vi "15.10.04 Interface+Data1.vi"() -> ()   [LabVIEW 2014]
panel:
  in  "NÚMERO DE CICLOS":dbl
  in  "Liga/Desliga":bool
  in  "Escolha: Porta Serial":refnum<visa-resource-name>="COM3"
  out "Dessorção":bool
  out "Adssorção":bool
  out "Single-Pass":bool
  out "Batch":bool
  in  "BATCH / SINGLE PASS":bool
  in  "Corrente":path
  in  "pH":path
  in  "Condutividade":path
  out "CORRENTE (A)":dbl(graph)
  out "pH":dbl(graph)
  out "CONDUTIVIDADE (us/cm)":dbl(graph)
  in  "?":enum32{"POTENCIOSTÁTICO", "GALVANOSTÁTICO"}(tab)
  in  "CONDUTIVIDADE \nMÁXIMA NA DESSORÇÃO P":dbl
  in  "TEMPO DE DESSOR敲O P":dbl
  in  "CONDUTIVIDADE \nMÍNIMA NA ADSORÇÃO P":dbl
  in  "TEMPO DE ADSOR敲O P":dbl
  in  "POTENCIAL DE CORTE\nNA DESSOR敲O (V) G":dbl
  in  "POTENCIAL DE CORTE\nNA ADSOR敲O (V) G":dbl
  in  "CONDUTIVIDADE \nMÍNIMA NA DESSORÇÃO G":dbl
  in  "TEMPO DE DESSOR敲O G":dbl
  in  "CONDUTIVIDADE \nMÍNIMA NA ADSORÇÃO G":dbl
  in  "TEMPO DE ADSOR敲O G":dbl
  # "s"
  # "us/cm"
  # "s"
  # "us/cm"
  # "s"
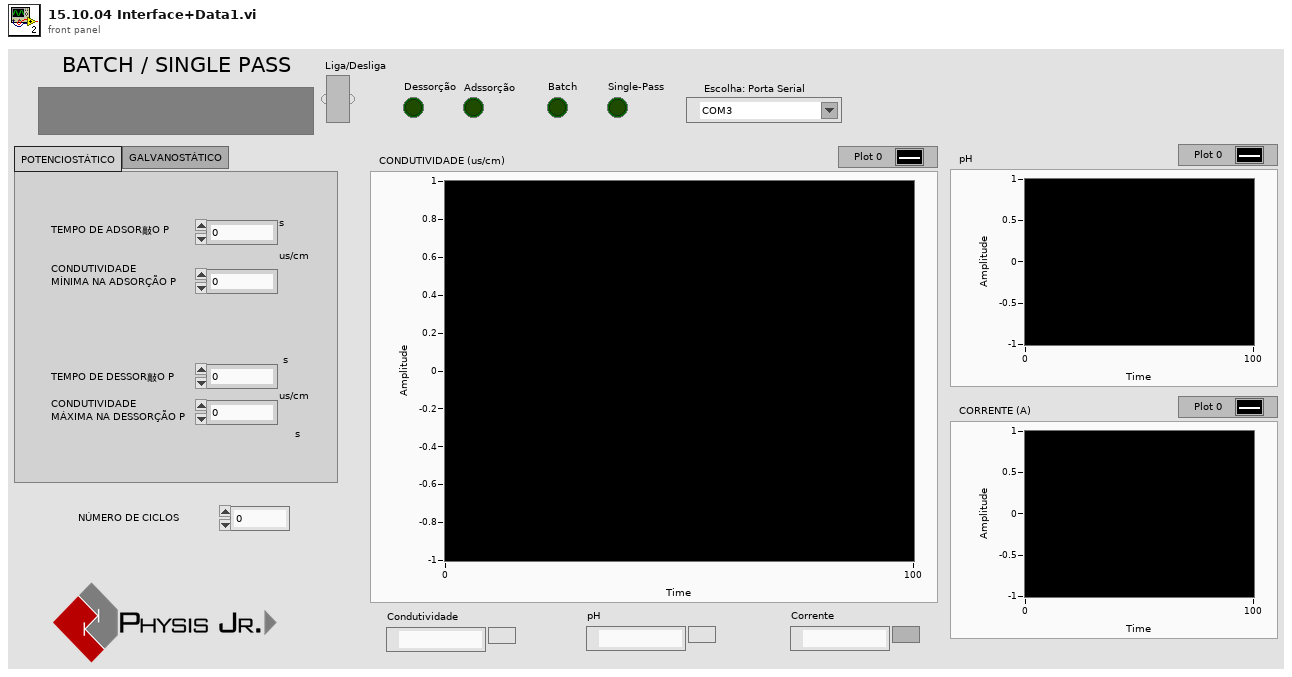
[diagram p1: front panel]
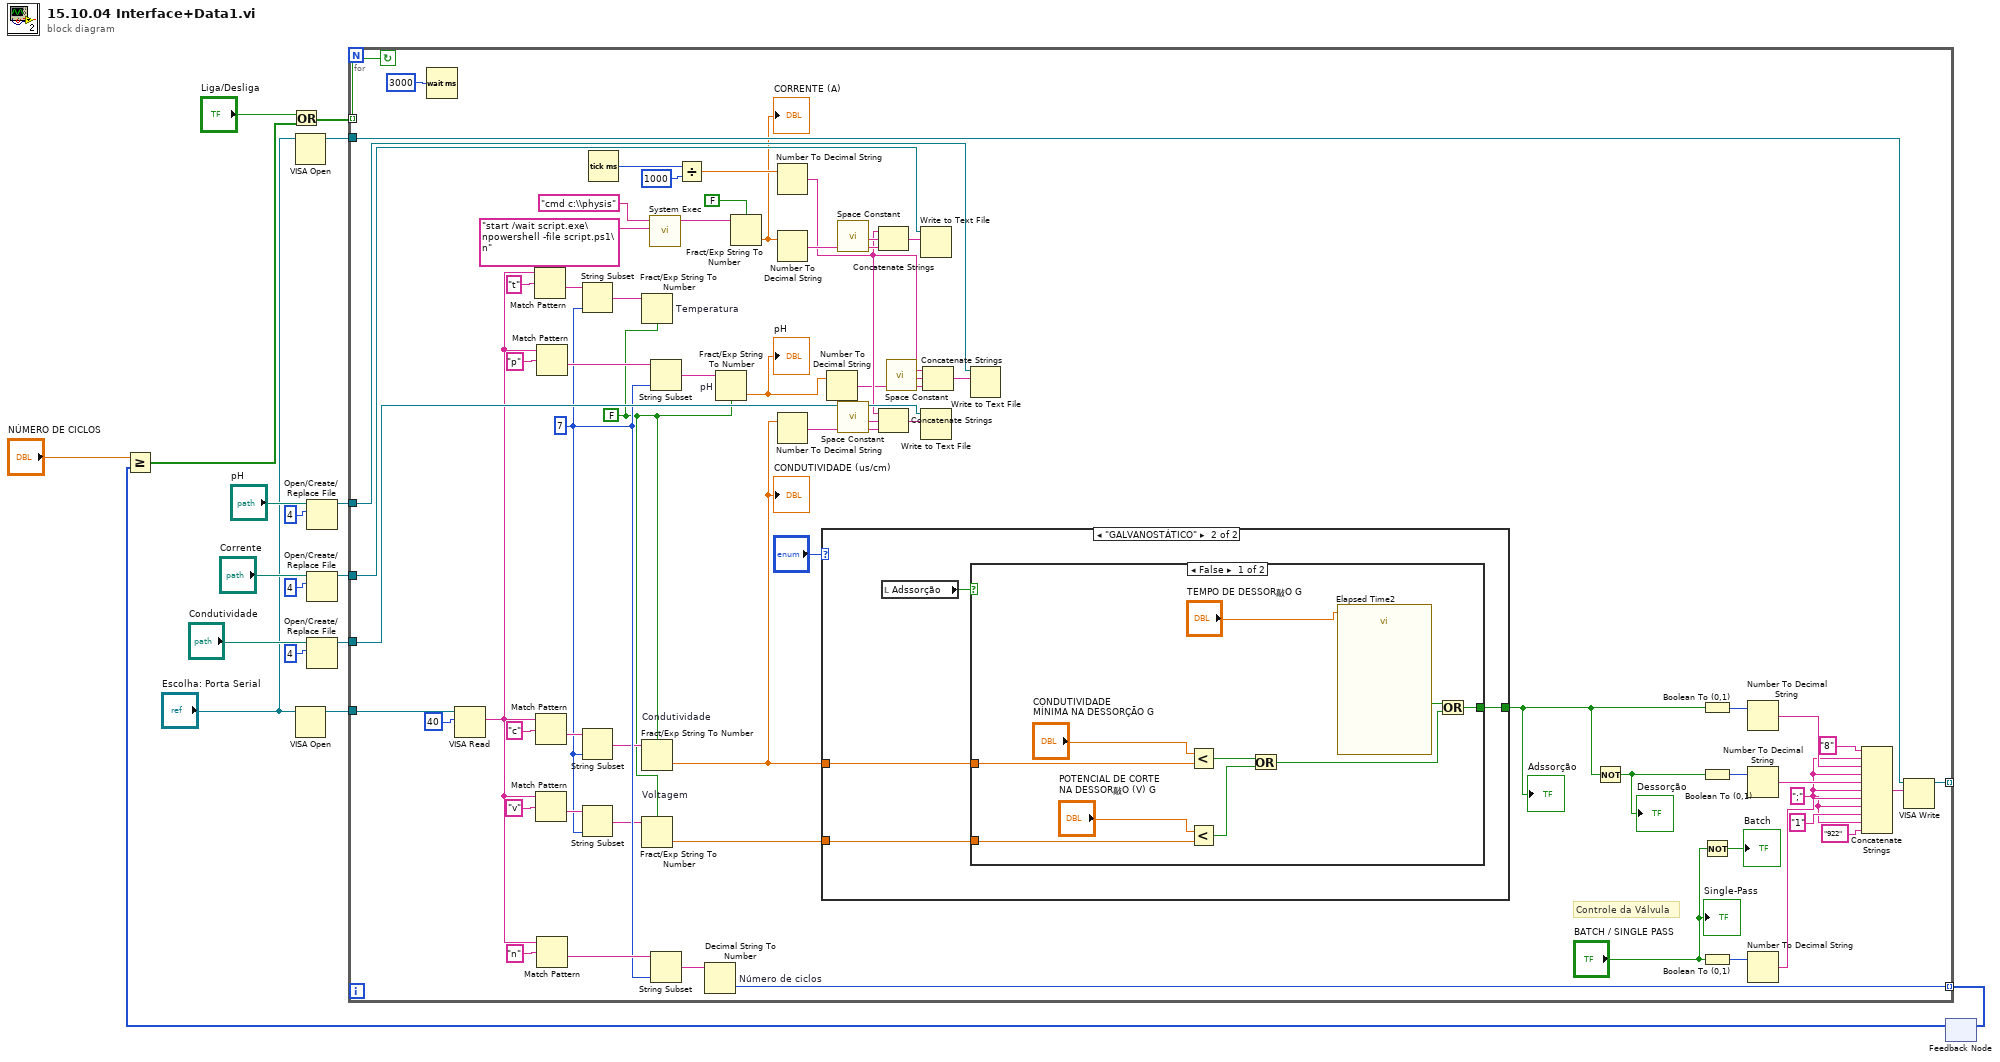
[diagram p0: block diagram]
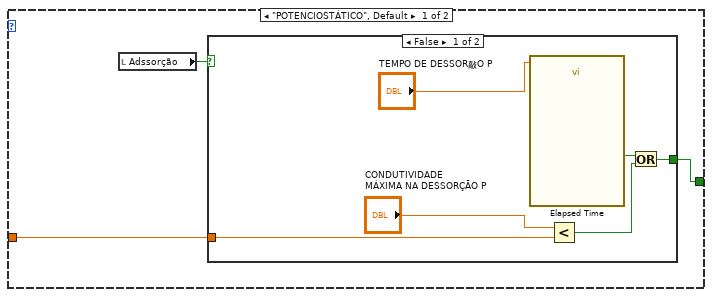
[diagram p2: hidden frame]
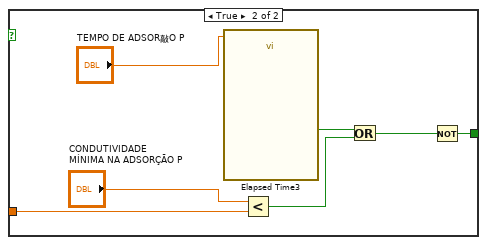
[diagram p3: hidden frame]
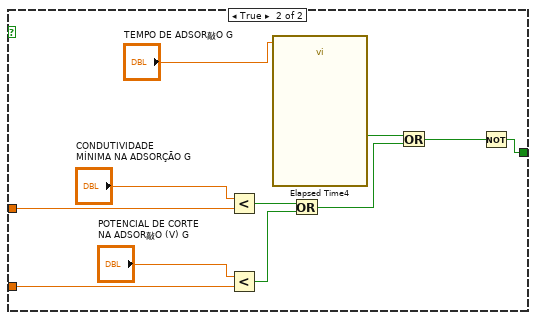
[diagram p4: hidden frame]
diagram:
  n1 = VISA Open(VISA resource name="Escolha: Porta Serial") -> (VISA resource name=w7:refnum<visa-resource-name>)  [unwired: 4 in, 1 out]
  n2 = VISA Open(VISA resource name="Escolha: Porta Serial") -> (VISA resource name=w9:refnum<visa-resource-name>)  [unwired: 4 in, 1 out]
  n3 = Open/Create/Replace File(file path (use dialog)="pH", operation (0:open)=4) -> (refnum out=w13:refnum<file>)  [unwired: 4 in, 2 out]
  n4 = Open/Create/Replace File(file path (use dialog)="Corrente", operation (0:open)=4) -> (refnum out=w11:refnum<file>)  [unwired: 4 in, 2 out]
  n5 = Open/Create/Replace File(file path (use dialog)="Condutividade", operation (0:open)=4) -> (refnum out=w17:refnum<file>)  [unwired: 4 in, 2 out]
  n6 = feedback #1() -> (w1:i32[])  [unwired: 1 in]
  n7 = Greater Or Equal?(x="NÚMERO DE CICLOS", y=w1) -> (x >= y?=w4:bool[])
  n8 = Or(x="Liga/Desliga", y=w4) -> (x .or. y?=w3:bool[])
  n9 = for {
    tunnel: w17 -> [w82]
    tunnel: w13 -> [w81]
    tunnel: w11 -> [w80]
    tunnel: w9 -> [w66]
    tunnel: w7 -> [w65]
    tunnel: [w64] -> _ mode=indexing
    tunnel: w3 -> [w63] mode=indexing
    tunnel: [w62] -> w2 mode=indexing
    stop <- w63 continue-if-true
    w32 = FALSE
    w38 = 7
    w69 = ";"
    # "Controle da Válvula"
    n10 = Wait (ms)(milliseconds to wait=3000) -> ()  [unwired: 1 out]
    n11 = VISA Read(VISA resource name=w66, byte count=40) -> (read buffer=w44:string)  [unwired: 1 in, 3 out]
    n12 = Match Pattern(string=w44, regular expression="t") -> (after substring=w42:string)  [unwired: 1 in, 3 out]
    n13 = Match Pattern(string=w44, regular expression="c") -> (after substring=w41:string)  [unwired: 1 in, 3 out]
    n14 = Match Pattern(string=w44, regular expression="v") -> (after substring=w40:string)  [unwired: 1 in, 3 out]
    n15 = Match Pattern(string=w44, regular expression="p") -> (after substring=w43:string)  [unwired: 1 in, 3 out]
    n16 = Match Pattern(string=w44, regular expression="n") -> (after substring=w39:string)  [unwired: 1 in, 3 out]
    n17 = String Subset(string=w42, length (rest)=w38) -> (substring=w36:string)  [unwired: 1 in]
    n18 = String Subset(string=w41, length (rest)=w38) -> (substring=w35:string)  [unwired: 1 in]
    n19 = String Subset(string=w40, length (rest)=w38) -> (substring=w34:string)  [unwired: 1 in]
    n20 = Tick Count (ms)() -> (millisecond timer value=w31:u32)
    n21 = Fract/Exp String To Number "Temperatura"(use system decimal point (T)=w32, string=w36) -> ()  [unwired: 2 in, 2 out]
    n22 = Fract/Exp String To Number "Condutividade"(use system decimal point (T)=w32, string=w35) -> (number=w20:dbl)  [unwired: 2 in, 1 out]
    "CONDUTIVIDADE (us/cm)" <- w20
    n23 = Fract/Exp String To Number "Voltagem"(use system decimal point (T)=w32, string=w34) -> (number=w19:dbl)  [unwired: 2 in, 1 out]
    n24 = call <vilib>:"System Exec.vi"("standard input"="start /wait script.exe\npowershell -file script.ps1\n", "command line"="cmd c:\\physis") -> ("standard output"=w24:string)  [unwired: 6 in, 3 out]
    n25 = String Subset(string=w43, length (rest)=w38) -> (substring=w37:string)  [unwired: 1 in]
    n26 = String Subset(string=w39, length (rest)=w38) -> (substring=w27:string)  [unwired: 1 in]
    n27 = Divide(x=w31, y=1000) -> (x/y=w29:dbl)
    n28 = Decimal String To Number "Número de ciclos"(string=w27) -> (number=w62:i32)  [unwired: 2 in, 1 out]
    n29 = Fract/Exp String To Number "pH"(use system decimal point (T)=w32, string=w37) -> (number=w33:dbl)  [unwired: 2 in, 1 out]
    "pH" <- w33
    n30 = Fract/Exp String To Number(use system decimal point (T)=FALSE, string=w24) -> (number=w23:dbl)  [unwired: 2 in, 1 out]
    "CORRENTE (A)" <- w23
    n31 = Number To Decimal String(number=w29) -> (decimal integer string=w52:string)  [unwired: 1 in]
    n32 = Number To Decimal String(number=w23) -> (decimal integer string=w53:string)  [unwired: 1 in]
    n33 = Number To Decimal String(number=w20) -> (decimal integer string=w59:string)  [unwired: 1 in]
    n34 = case shown="\"GALVANOSTÁTICO\"" "?" {
      tunnel: [w85 w102] -> w61
      tunnel: w20 -> [w84 w101]
      tunnel: w19 -> [_ w100]
      frame "POTENCIOSTÁTICO", Default {
        n35 = local read "Adssorção"() -> (w86:bool)
        n36 = case shown="False" w86 {
          tunnel: [w91 w98] -> w85
          tunnel: w84 -> [w89 w95]
          frame False {
            n37 = call "Elapsed Time"("Time Target (s)"="TEMPO DE DESSOR敲O P") -> ("Time has Elapsed"=w87:bool)  [unwired: 11 in, 7 out]
            n38 = Less?(x="CONDUTIVIDADE \nMÁXIMA NA DESSORÇÃO P", y=w89) -> (x < y?=w90:bool)
            n39 = Or(x=w87, y=w90) -> (x .or. y?=w91:bool)
          }
          frame True {
            n40 = call "Elapsed Time3"("Time Target (s)"="TEMPO DE ADSOR敲O P") -> ("Time has Elapsed"=w93:bool)  [unwired: 11 in, 7 out]
            n41 = Less?(x="CONDUTIVIDADE \nMÍNIMA NA ADSORÇÃO P", y=w95) -> (x < y?=w96:bool)
            n42 = Or(x=w93, y=w96) -> (x .or. y?=w97:bool)
            n43 = Not(x=w97) -> (.not. x?=w98:bool)
          }
        }
      }
      frame "GALVANOSTÁTICO" {
        n44 = local read "Adssorção"() -> (w103:bool)
        n45 = case shown="False" w103 {
          tunnel: [w111 w123] -> w102
          tunnel: w101 -> [w107 w115]
          tunnel: w100 -> [w104 w114]
          frame False {
            n46 = Less?(x="CONDUTIVIDADE \nMÍNIMA NA DESSORÇÃO G", y=w107) -> (x < y?=w108:bool)
            n47 = Less?(x="POTENCIAL DE CORTE\nNA DESSOR敲O (V) G", y=w104) -> (x < y?=w109:bool)
            n48 = Or(x=w108, y=w109) -> (x .or. y?=w110:bool)
            n49 = call "Elapsed Time2"("Time Target (s)"="TEMPO DE DESSOR敲O G") -> ("Time has Elapsed"=w105:bool)  [unwired: 11 in, 7 out]
            n50 = Or(x=w105, y=w110) -> (x .or. y?=w111:bool)
          }
          frame True {
            n51 = Less?(x="CONDUTIVIDADE \nMÍNIMA NA ADSORÇÃO G", y=w115) -> (x < y?=w120:bool)
            n52 = Less?(x="POTENCIAL DE CORTE\nNA ADSOR敲O (V) G", y=w114) -> (x < y?=w118:bool)
            n53 = call "Elapsed Time4"("Time Target (s)"="TEMPO DE ADSOR敲O G") -> ("Time has Elapsed"=w116:bool)  [unwired: 11 in, 7 out]
            n54 = Or(x=w120, y=w118) -> (x .or. y?=w119:bool)
            n55 = Or(x=w116, y=w119) -> (x .or. y?=w124:bool)
            n56 = Not(x=w124) -> (.not. x?=w123:bool)
          }
        }
      }
    }
    "Adssorção" <- w61
    n57 = Number To Decimal String(number=w33) -> (decimal integer string=w51:string)  [unwired: 1 in]
    n58 = call <vilib>:"Space Constant.vi"() -> ("String"=w56:string)
    n59 = call <vilib>:"Space Constant.vi"() -> ("String"=w60:string)
    n60 = Concatenate Strings(w52, w56, w53) -> (w57:string)
    n61 = Concatenate Strings(w52, w60, w59) -> (w58:string)
    n62 = call <vilib>:"Space Constant.vi"() -> ("String"=w55:string)
    n63 = Write to Text File(file (use dialog)=w80, text=w57) -> ()  [unwired: 2 in, 3 out]
    n64 = Write to Text File(file (use dialog)=w82, text=w58) -> ()  [unwired: 2 in, 3 out]
    n65 = Concatenate Strings(w52, w55, w51) -> (w54:string)
    n66 = Write to Text File(file (use dialog)=w81, text=w54) -> ()  [unwired: 2 in, 3 out]
    n67 = Not(x=w61) -> (.not. x?=w78:bool)
    "Dessorção" <- w78
    n68 = Boolean To (0,1)(Boolean=w61) -> (0, 1=w75:i16)
    n69 = Boolean To (0,1)(Boolean=w78) -> (0, 1=w74:i16)
    n70 = Not(x="BATCH / SINGLE PASS") -> (.not. x?=→"Batch":bool)
    n71 = Boolean To (0,1)(Boolean="BATCH / SINGLE PASS") -> (0, 1=w76:i16)
    n72 = Number To Decimal String(number=w75) -> (decimal integer string=w73:string)  [unwired: 1 in]
    n73 = Number To Decimal String(number=w74) -> (decimal integer string=w72:string)  [unwired: 1 in]
    n74 = Number To Decimal String(number=w76) -> (decimal integer string=w71:string)  [unwired: 1 in]
    n75 = Concatenate Strings("8", w69, w73, w69, w72, w69, w71, w69, "1", w69, "922") -> (w67:string)
    n76 = VISA Write(VISA resource name=w65, write buffer=w67) -> (VISA resource name out=w64:refnum<visa-resource-name>)  [unwired: 1 in, 2 out]
    "Single-Pass" <- "BATCH / SINGLE PASS"
  }
  n77 = feedback-in #1(w2) -> ()
